vi "Nonlinear Curve Fit TRDL bound.vi"(0 "Y":dbl[](array[numeric]), 1 "f(x,a)":T3, 2 "data":variant, 5 "X":dbl[](array[numeric]), 7 "Weight":dbl[](array[numeric]), 9 "initial parameters":dbl[](array[numeric]), 11 "error in (no error)":errorcluster, 12 "termination":cluster{"max iteration":i32, "tolerance":dbl}={"max iteration"=200, "tolerance"=1e-08}, 13 "parameter bounds":T2, 14 "method":T1 items=["Least Square", "Least Absolute Residual", "Bisquare"]) -> (3 "number of function calls":i32, 4 "best nonlinear fit":dbl[](array[numeric]), 6 "best fit parameters":dbl[](array[numeric]), 8 "covariance":T4, 10 "residue":dbl, 15 "error out":errorcluster)   [LabVIEW 2014, in "NI_Gmath.lvlib"]
doc: "Uses either the Levenberg-Marquardt algorithm or the trust-region dogleg algorithm to determine the set of parameters that best fit the set of input data points (<B>X</B>, <B>Y</B>) as expressed by a nonlinear function y = <B>f(x,a)</B>, where a is the set of parameters. You must manually select the polymorphic instance to use."
uses:
  NI_Gmath.lvlib
  RealMatrix.ctl
  LM model function reference.ctl
  Curve Fitting Criteria.ctl
  stopping criteria.ctl
  LM model function.ctl
  LM_output select.ctl
  Real Inverse Matrix.vi
  NI_AALBase.lvlib
  NI_Matrix.lvlib
  NI_AALPro.lvlib
panel:
  in  "TR update constants":cluster{"h1":dbl, "h2":dbl, "a1":dbl, "a2":dbl}={"h1"=0.0001, "h2"=0.99, "a1"=0.25, "a2"=3.5}
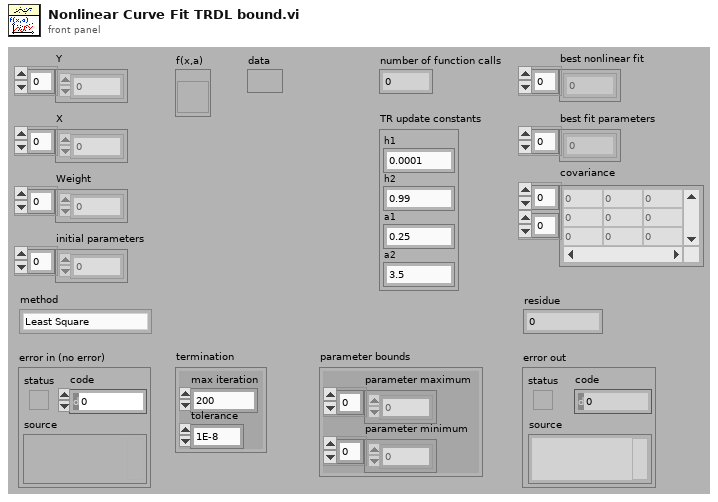
[diagram p1: front panel]
types:
  T1 = typedef "NI_AALPro.lvlib/Curve Fitting Criteria.ctl" = u16
  T2 = cluster{"parameter minimum":dbl[], "parameter maximum":dbl[]}
  T3 = typedef "NI_Gmath.lvlib/LM model function reference.ctl" = refnum<vi>
  T4 = typedef "NI_Matrix.lvlib/RealMatrix.ctl" = dbl[][]
  T5 = typedef "NI_Gmath.lvlib/LM model function.ctl" = cluster{"f(x,a)":T3, "data":variant}
  T6 = typedef "NI_Gmath.lvlib/stopping criteria.ctl" = cluster{"function tolerance":dbl, "parameter tolerance":dbl, "max iterations":i32, "max function calls":i32, "gradient tolerance":dbl, "max time (sec)":dbl}
  T7 = typedef "NI_Gmath.lvlib/stopping criteria with time.ctl" = cluster{"function tolerance":dbl, "parameter tolerance":dbl, "max iterations":i32, "max function calls":i32, "gradient tolerance":dbl, "max time (sec)":dbl, "initial tick count":u32}
  T8 = typedef "NI_Gmath.lvlib/LM_output select.ctl" = cluster{"model function":bool, "gradient":bool}
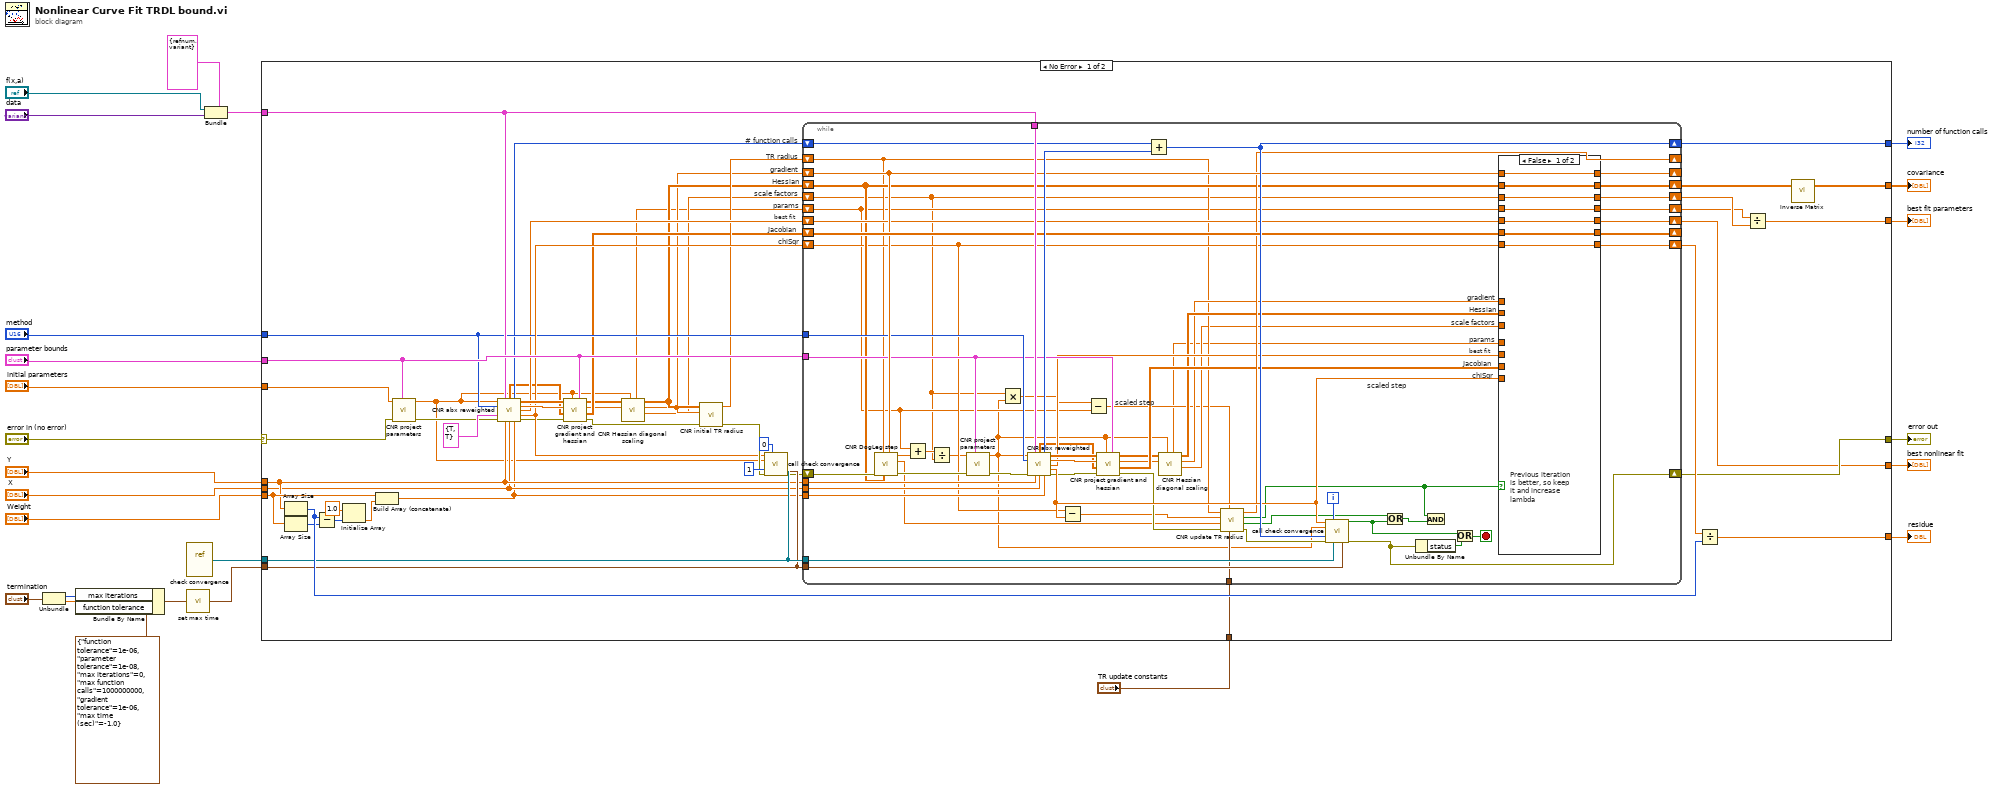
[diagram p0: block diagram]
diagram:
  n1 = Unbundle("termination") -> ("max iteration"=w13:i32, "tolerance"=w1:dbl)
  n2 = Bundle By Name(cluster=T6 {"function tolerance"=1e-06, "parameter tolerance"=1e-08, "max iterations"=0, "max function calls"=1000000000, "gradient tolerance"=1e-06, "max time (sec)"=-1.0} ("stopping criteria"), "max iterations"=w13, "function tolerance"=w1) -> (w7:T6)
  n3 = vi-ref "check convergence.vi"() -> (w12:refnum<vi>)
  n4 = call "set max time.vi"("stopping criteria"=w7) -> ("stopping criteria"=w6:T7)
  n5 = Bundle(cluster=T5 {"f(x,a)"=refnum, "data"=variant} ("model function"), "f(x,a)"="f(x,a)", "data"="data") -> (w8:T5)
  n6 = case shown="No Error" "error in (no error)" {
    selector: "error in (no error)" -> [w56 w152]
    tunnel: [w26 _] -> w25
    tunnel: [w71 _] -> w24
    tunnel: "initial parameters" -> [w30 _]
    tunnel: [w40 _] -> w22
    tunnel: [w57 _] -> w21
    tunnel: "Weight" -> [w66 _]
    tunnel: "Y" -> [w44 _]
    tunnel: w6 -> [w73 _]
    tunnel: "X" -> [w43 _]
    tunnel: [w61 w152] -> w17
    tunnel: w8 -> [w50 _]
    tunnel: w12 -> [w74 _]
    tunnel: [w62 _] -> w11
    tunnel: "parameter bounds" -> [w55 _]
    tunnel: "method" -> [w49 _]
    tunnel: "TR update constants" -> [w39 _]
    frame No Error {
      # "# function calls"
      # "gradient"
      # "Hessian"
      # "scale factors"
      # "TR radius"
      # "Jacobian"
      # "best fit"
      # "chiSqr"
      # "params"
      n7 = Array Size(array=w44) -> (size(s)=w75:i32)
      n8 = Array Size(array=w66) -> (size(s)=w69:i32)
      n9 = Subtract(x=w75, y=w69) -> (x-y=w68:i32)
      n10 = Initialize Array(1.0, w68) -> (w67:dbl[])
      n11 = Build Array (concatenate)(w66, w67) -> (w42:dbl[])
      n12 = call "CNR project parameters.vi"("bounds"=w55, "error in"=w56, "parameters"=w30) -> ("error out"=w48:errorcluster, "projected parameters"=w29:dbl[])  [unwired: 7 out]
      n13 = call "CNR abx reweighted.vi"("parameters"=w29, "model function"=w50, "method"=w49, "output control"=T8 {"model function"=TRUE, "gradient"=TRUE}, "error in (no error)"=w48, "Y"=w44, "X"=w43, "Weight"=w42) -> ("Jacobian"=w37:T4, "number of function calls"=w47:i32, "Hessian"=w54:T4, "gradient"=w53:dbl[], "best fit"=w41:dbl[], "chiSqr"=w52:dbl, "error out"=w46:errorcluster)  [unwired: 1 in]
      n14 = call "CNR project gradient and hessian.vi"("bounds"=w55, "projected parameters"=w29, "error in"=w46, "Jacobian"=w37, "gradient"=w53, "Hessian"=w54) -> ("error out"=w45:errorcluster, "projected jacobian"=w36:T4, "projected gradient"=w33:dbl[], "projected Hessian"=w35:T4)  [unwired: 1 in, 1 out]
      n15 = call "CNR Hessian diagonal scaling.vi"("parameters"=w29, "gradient"=w33, "Hessian"=w35) -> ("D"=w31:dbl[], "scaled gradient"=w32:dbl[], "scaled Hessian"=w34:T4, "scaled parameters"=w28:dbl[])  [unwired: 5 out]
      n16 = call "CNR initial TR radius.vi"("error in"=w45, "g"=w32, "H"=w34) -> ("error out"=w59:errorcluster, "initial TR radius"=w38:dbl)  [unwired: 7 out]
      n17 = call "call check convergence.vi"("f"=w52, "current iteration"=0, "X"=w29, "number of function evaluations"=1, "error in"=w59, "vi reference"=w74, "stopping criteria"=w73) -> ("error out"=w65:errorcluster)  [unwired: 1 in, 7 out]
      n18 = while {
        tunnel: w43 -> [w136]
        tunnel: w44 -> [w104]
        shift-left: w52 -> [w98]
        shift-right: [w127] -> w72
        shift-left: w28 -> [w85]
        shift-right: [w120] -> w27
        shift-left: w38 -> [w86]
        shift-right: [w105] -> _
        shift-right: [w123] -> w61
        shift-left: w65 -> [w125]
        tunnel: w50 -> [w135]
        tunnel: w74 -> [w130]
        tunnel: w73 -> [w129]
        shift-right: [w131] -> w62
        shift-left: w47 -> [w134]
        shift-right: [w133] -> w40
        shift-left: w41 -> [w103]
        shift-right: [w128] -> _
        shift-left: w36 -> [w119]
        tunnel: w42 -> [w113]
        shift-right: [w118] -> w60
        shift-left: w31 -> [w77]
        tunnel: w55 -> [w106]
        shift-right: [w117] -> _
        shift-left: w32 -> [w115]
        shift-right: [w116] -> w58
        shift-left: w34 -> [w100]
        tunnel: w49 -> [w114]
        tunnel: w39 -> [w101]
        i -> [w132]
        stop <- w121 stop-if-true
        # "scaled step"
        # "scaled step"
        # "chiSqr"
        # "Jacobian"
        # "best fit"
        # "params"
        # "scale factors"
        # "Hessian"
        # "gradient"
        n19 = call "CNR DogLeg step.vi"("gradient"=w115, "Hessian"=w100, "TR radius"=w86, "error in (no error)"=w125) -> ("error out"=w112:errorcluster, "L(0)-L(hdl)\npredicted change"=w91:dbl, "x step"=w83:dbl[])  [unwired: 3 in, 2 out]
        n20 = Add(x=w85, y=w83) -> (x+y=w82:dbl[])
        n21 = Divide(x=w82, y=w77) -> (x/y=w81:dbl[])
        n22 = call "CNR project parameters.vi"("bounds"=w106, "error in"=w112, "parameters"=w81) -> ("error out"=w111:errorcluster, "projected parameters"=w78:dbl[])  [unwired: 7 out]
        n23 = Multiply(x=w77, y=w78) -> (x*y=w76:dbl[])
        n24 = call "CNR abx reweighted.vi"("parameters"=w78, "model function"=w135, "method"=w114, "error in (no error)"=w111, "Y"=w104, "X"=w136, "Weight"=w113) -> ("Jacobian"=w89:T4, "number of function calls"=w137:i32, "Hessian"=w108:T4, "gradient"=w107:dbl[], "best fit"=w102:dbl[], "chiSqr"=w124:dbl, "error out"=w110:errorcluster)  [unwired: 2 in]
        n25 = Subtract(x=w98, y=w124) -> (x-y=w92:dbl)
        n26 = Subtract(x=w76, y=w85) -> (x-y=w80:dbl[])
        n27 = call "CNR project gradient and hessian.vi"("bounds"=w106, "projected parameters"=w78, "error in"=w110, "Jacobian"=w89, "gradient"=w107, "Hessian"=w108) -> ("error out"=w109:errorcluster, "projected jacobian"=w99:T4, "projected gradient"=w94:dbl[], "projected Hessian"=w96:T4)  [unwired: 1 in, 1 out]
        n28 = Add(x=w134, y=w137) -> (x+y=w131:i32)
        n29 = call "CNR Hessian diagonal scaling.vi"("parameters"=w78, "gradient"=w94, "Hessian"=w96) -> ("D"=w84:dbl[], "scaled gradient"=w93:dbl[], "scaled Hessian"=w95:T4, "scaled parameters"=w79:dbl[])  [unwired: 5 out]
        n30 = call "CNR update TR radius.vi"("TR update constants"=w101, "step"=w80, "error in (no error)"=w109, "L(0)-L(p_dl)"=w91, "F(x)-F(x+p)"=w92, "TR Radius"=w86) -> ("error out"=w126:errorcluster, "quit?"=w90:bool, "step OK?"=w97:bool, "TR Radius out"=w105:dbl)  [unwired: 2 out]
        n31 = call "call check convergence.vi"("f"=w124, "current iteration"=w132, "X"=w78, "number of function evaluations"=w131, "error in"=w126, "vi reference"=w130, "stopping criteria"=w129) -> ("stop?"=w87:bool, "error out"=w123:errorcluster)  [unwired: 1 in, 6 out]
        n32 = Or(x=w90, y=w87) -> (x .or. y?=w88:bool)
        n33 = Unbundle By Name(w123) -> ("status"=w122:bool)
        n34 = And(x=w97, y=w88) -> ()  [unwired: 1 out]
        n35 = Or(x=w87, y=w122) -> (x .or. y?=w121:bool)
        n36 = case shown="False" w97 {
          tunnel: w79 -> [_ w145]
          tunnel: w85 -> [w144 _]
          tunnel: [w144 w145] -> w120
          tunnel: w98 -> [w143 _]
          tunnel: w124 -> [_ w151]
          tunnel: [w143 w151] -> w127
          tunnel: w103 -> [w142 _]
          tunnel: [w142 w149] -> w133
          tunnel: w119 -> [w141 _]
          tunnel: [w141 w150] -> w128
          tunnel: w99 -> [_ w150]
          tunnel: w102 -> [_ w149]
          tunnel: w77 -> [w140 _]
          tunnel: [w140 w146] -> w118
          tunnel: w115 -> [w139 _]
          tunnel: w100 -> [w138 _]
          tunnel: [w139 w148] -> w117
          tunnel: [w138 w147] -> w116
          tunnel: w93 -> [_ w148]
          tunnel: w95 -> [_ w147]
          tunnel: w84 -> [_ w146]
          frame False {
            # "Previous iteration\nis better, so keep\nit and increase \nlambda"
          }
          frame True {
            # "Current iteration\nis better, so use\nit and decrease \nlambda"
          }
        }
      }
      n37 = Divide(x=w72, y=w75) -> (x/y=w71:dbl)
      n38 = Divide(x=w27, y=w60) -> (x/y=w26:dbl[])
      n39 = call-poly "Inverse Matrix.vi"("Input Matrix"=w58) -> ("Inverse Matrix"=w57:T4)  [unwired: 1 in, 1 out]
    }
    frame Error {
    }
  }
  "residue" <- w24
  "best fit parameters" <- w25
  "best nonlinear fit" <- w22
  "error out" <- w17
  "covariance" <- w21
  "number of function calls" <- w11
